vi "INIT shooter.vi"(8 "error in (no error)":errorcluster) -> (0 "error out":errorcluster)   [LabVIEW 2023]
uses:
  Global INIT.vi
  <vilib>/Rock Robotics/WPI/ThirdParty/REV Robotics/REVLib/SubVI/Public/SPARK Configure Basic Ramp Rate.vi
  <vilib>/Rock Robotics/WPI/ThirdParty/REV Robotics/REVLib/SubVI/Public/SPARK Configure Follower Mode From Ref.vi
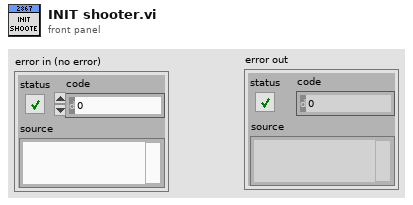
[diagram p1: front panel]
types:
  T1 = typedef "ctrl swerve motor.ctl" = cluster{"description":string, "MOTOR SELECT":T2, "Installed?":bool, "CAN ID":u8, "refnum name":string, "Invert":bool, "Idle Mode":T3, "Current limiting":T4, "MOTOR PIDF coefficients":T5, "gear ratio":dbl}
  T2 = typedef "ctrl MOTOR SELECT.ctl" = i16
  T3 = typedef "Spark MAX Idle Mode.ctl" = enum16{"Coast", "Brake"}
  T4 = typedef "ctrl Spark MAX current limiting.ctl" = cluster{"Linearized":bool, "Free Speed (A)":dbl, "Primay (A)":dbl, "Limit RPM (0)":u32}
  T5 = typedef "ctrl motor PIDF coefficients.ctl" = cluster{"PIDF":cluster{"P Gain":dbl, "I Gain":dbl, "D Gain":dbl, "F Gain":dbl, "I Zone":dbl, "Min Output":dbl, "Max Output":dbl}, "Smart Motion":T6}
  T6 = typedef "Spark MAX Smart Motion Parameters.ctl" = cluster{"Max Velocity":dbl, "Max Acceleration":dbl, "Minimum Velocity Output":dbl, "Allowed Closed Loop Error":dbl}
  T7 = typedef "WPI_MotorControlDeviceRef.ctl" = cluster{"DeviceStatus":errorcluster, "Type":T8, "PWM":cluster{"PWM Channel":T9, "DeadBand":T10}, "CAN":cluster{"Device Number":u8, "SetOutput VI Ref":variant, "GetOutput VI Ref":variant, "Enable VI Ref":variant, "Disable VI Ref":variant, "Data":variant}, "Invert":bool, "DIO PWM":cluster{"PWM \"Enable\" Channel":T9, "DIOChannel":T11, "PWM Rate":dbl}}
  T8 = typedef "WPI_MotorControlType.ctl" = enum16{"PWM", "CAN", "DIO PWM"}
  T9 = typedef "FPGA_DIOPWMChannel.ctl" = enum8{"PWM 0", "PWM 1", "PWM 2", "PWM 3", "PWM 4", "PWM 5", "PWM 6", "PWM 7", "PWM 8", "PWM 9", "PWM MXP 0", "PWM MXP 1", "PWM MXP 2", "PWM MXP 3", "PWM MXP 4", "PWM MXP 5", "PWM MXP 6", "PWM MXP 7", "PWM MXP 8", "PWM MXP 9", "Invalid"}
  T10 = typedef "WPI_PWMDeadband.ctl" = cluster{"Name":string, "maxPositivePwm":i32, "minPositivePwm":i32, "centerPwm":i32, "maxNegativePwm":i32, "minNegativePwm":i32, "angularRange":u16}
  T11 = typedef "FPGA_DIOChannel.ctl" = enum8{"DIO 0", "DIO 1", "DIO 2", "DIO 3", "DIO 4", "DIO 5", "DIO 6", "DIO 7", "DIO 8", "DIO 9", "DIO MXP 0", "DIO MXP 1", "DIO MXP 2", "DIO MXP 3", "DIO MXP 4", "DIO MXP 5", "DIO MXP 6", "DIO MXP 7", "DIO MXP 8", "DIO MXP 9", "DIO MXP 10", "DIO MXP 11", "DIO MXP 12", "DIO MXP 13", "DIO MXP 14", "DIO MXP 15", "SPI Port CS1", "SPI Port CS2", "SPI Port CS3", "SPI Port MISO", "SPI Port MOSI", "Invalid"}
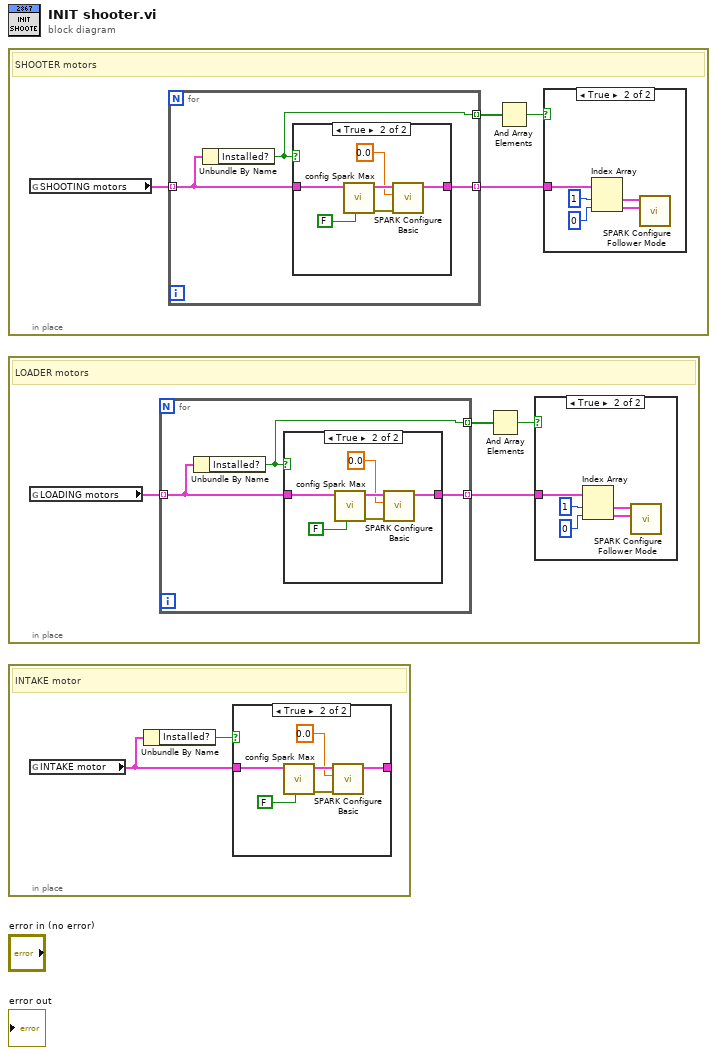
[diagram p0: block diagram]
diagram:
  n1 = in-place {
    # "SHOOTER motors"
    n2 = global read "Global INIT.vi" "SHOOTING motors"() -> (w4:T1[])
    n3 = for {
      tunnel: w4 -> [w12] mode=indexing
      tunnel: [w11] -> w3 mode=indexing
      tunnel: [w10] -> w1 mode=indexing
      n4 = Unbundle By Name(w12) -> ("Installed?"=w11:bool)
      n5 = case shown="True" w11 {
        tunnel: w12 -> [_ w16]
        tunnel: [_ w13] -> w10
        frame False {
        }
        frame True {
          n6 = call "config Spark Max.vi"("LIMIT SW\nEnabled?"=FALSE ("LIMIT SW\nEnabled? (T)"), "motor\ndefaults"=w16) -> ("error out"=w18:errorcluster, "MotorControlDevRef"=w17:T7)  [unwired: 8 in]
          n7 = call-poly <vilib>:"SPARK Configure Basic.vi"("error in (no error)"=w18, "Seconds from neutral to full (0)"=sgl 0.0, "MotorControlDeviceRef in"=w17) -> ("MotorControlDeviceRef"=w13:T7)  [unwired: 7 in, 1 out]
        }
      }
    }
    n8 = And Array Elements(Boolean array=w3) -> (logical AND=w2:bool)
    n9 = case shown="True" w2 {
      tunnel: w1 -> [_ w9]
      frame False {
      }
      frame True {
        n10 = Index Array(array=w9, index #1=1 ("index"), index #2=0 ("index")) -> (element #1=w5:T7, element #2=w6:T7)
        n11 = call-poly <vilib>:"SPARK Configure Follower Mode.vi"("Leader MotorControlDeviceRef"=w6, "MotorControlDeviceRef in"=w5) -> ()  [unwired: 8 in, 2 out]
      }
    }
  }
  n12 = in-place {
    # "LOADER motors"
    n13 = global read "Global INIT.vi" "LOADING motors"() -> (w22:T1[])
    n14 = for {
      tunnel: w22 -> [w30] mode=indexing
      tunnel: [w29] -> w21 mode=indexing
      tunnel: [w28] -> w19 mode=indexing
      n15 = Unbundle By Name(w30) -> ("Installed?"=w29:bool)
      n16 = case shown="True" w29 {
        tunnel: w30 -> [_ w34]
        tunnel: [_ w31] -> w28
        frame False {
        }
        frame True {
          n17 = call "config Spark Max.vi"("LIMIT SW\nEnabled?"=FALSE ("LIMIT SW\nEnabled? (T)"), "motor\ndefaults"=w34) -> ("error out"=w36:errorcluster, "MotorControlDevRef"=w35:T7)  [unwired: 8 in]
          n18 = call-poly <vilib>:"SPARK Configure Basic.vi"("error in (no error)"=w36, "Seconds from neutral to full (0)"=sgl 0.0, "MotorControlDeviceRef in"=w35) -> ("MotorControlDeviceRef"=w31:T7)  [unwired: 7 in, 1 out]
        }
      }
    }
    n19 = And Array Elements(Boolean array=w21) -> (logical AND=w20:bool)
    n20 = case shown="True" w20 {
      tunnel: w19 -> [_ w27]
      frame False {
      }
      frame True {
        n21 = Index Array(array=w27, index #1=1 ("index"), index #2=0 ("index")) -> (element #1=w23:T7, element #2=w24:T7)
        n22 = call-poly <vilib>:"SPARK Configure Follower Mode.vi"("Leader MotorControlDeviceRef"=w24, "MotorControlDeviceRef in"=w23) -> ()  [unwired: 8 in, 2 out]
      }
    }
  }
  n23 = in-place {
    # "INTAKE motor"
    n24 = global read "Global INIT.vi" "INTAKE motor"() -> (w38:T1)
    n25 = Unbundle By Name(w38) -> ("Installed?"=w37:bool)
    n26 = case shown="True" w37 {
      tunnel: w38 -> [_ w42]
      tunnel: [_ w39] -> _
      frame False {
      }
      frame True {
        n27 = call "config Spark Max.vi"("LIMIT SW\nEnabled?"=FALSE ("LIMIT SW\nEnabled? (T)"), "motor\ndefaults"=w42) -> ("error out"=w44:errorcluster, "MotorControlDevRef"=w43:T7)  [unwired: 8 in]
        n28 = call-poly <vilib>:"SPARK Configure Basic.vi"("error in (no error)"=w44, "Seconds from neutral to full (0)"=sgl 0.0, "MotorControlDeviceRef in"=w43) -> ("MotorControlDeviceRef"=w39:T7)  [unwired: 7 in, 1 out]
      }
    }
  }
